vi "CreatePublicEvents.vi"(8 "error in (no error)":errorcluster, 11 "Setting Database":refnum<class "Setting Database.lvclass">) -> (0 "error out":errorcluster, 3 "Setting Database out":refnum<class "Setting Database.lvclass">)   [LabVIEW 2019, in "Setting Database.lvclass"]
doc: "---------------------------------------------------------------\nJKI State Machine Objects™\nhttp://jki.net/state-machine-objects/\nCopyright (C) 2005-2015, JKI <info@jki.net>\nALL RIGHTS RESERVEDJKI State Machine Objects (SMO) 1.0.0.4\nJKI - JKI\nCopyright (c) 2015, JKI"
uses:
  Setting Database.lvclass
  Typedefs/PublicEvents--Setting Database.NewActivePath.ctl
  Path Settings/Path Settings.lvclass
  Typedefs/PublicEvents--Setting Database.NewActiveRectangle.ctl
  Rectangle Settings/Rectangle Settings.lvclass
  Typedefs/PublicEvents--Setting Database.NewActiveFunnel.ctl
  Funnel Settings/Funnel Settings.lvclass
  Typedefs/PublicEvents--Setting Database.NewActiveDot.ctl
  Dot Settings/Dot Settings.lvclass
  Typedefs/PublicEvents--Setting Database.DotsUpdatedCheck.ctl
  Typedefs/PublicEvents--Setting Database.DotsUpdated.ctl
  Typedefs/PublicEvents--Setting Database.FunnelsUpdatedCheck.ctl
  Typedefs/PublicEvents--Setting Database.FunnelsUpdated.ctl
  Typedefs/PublicEvents--Setting Database.PathsUpdatedCheck.ctl
  Typedefs/PublicEvents--Setting Database.PathsUpdated.ctl
  Typedefs/PublicEvents--Setting Database.RectanglesUpdatedCheck.ctl
  Typedefs/PublicEvents--Setting Database.RectanglesUpdated.ctl
  Setting Database.lvclass/Setting Database.ctl
  <vilib>/JKI/JKI SMO/SMO/SMO.lvclass
panel:
  # "For instructions on how to use the JKI State Machine Objects, examples and video tutorials, visit:\nhttp://jki.net/state-machine-objects/\n\nJKI State Machine Objects™\nhttp://jki.net/state-machine-objects/\nCopyright (C) 2005-2015, JKI <info@jki.net>\nALL RIGHTS RESERVED"
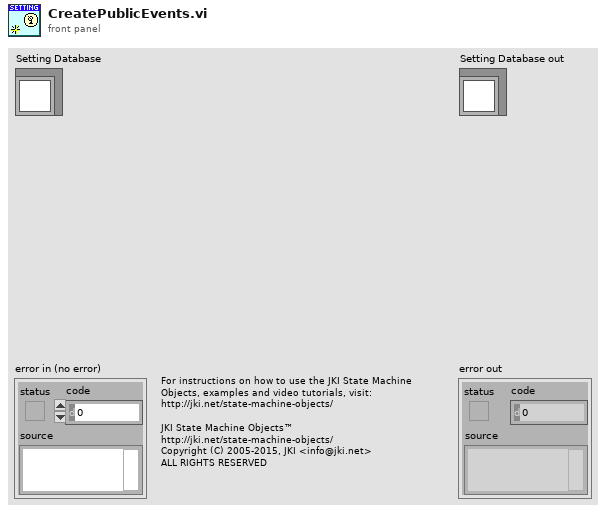
[diagram p1: front panel]
types:
  T1 = typedef "Setting Database.lvclass/PublicEvents--Setting Database.RectanglesUpdatedCheck.ctl" = cluster{"Read?":refnum<notifier>, "RectanglesUpdated":T2}
  T2 = typedef "Setting Database.lvclass/PublicEvents--Setting Database.RectanglesUpdated.ctl" = refnum<class "Rectangle Settings.lvclass">[]
  T3 = typedef "Setting Database.lvclass/PublicEvents--Setting Database.PathsUpdatedCheck.ctl" = cluster{"Read?":refnum<notifier>, "PathsUpdated":T4}
  T4 = typedef "Setting Database.lvclass/PublicEvents--Setting Database.PathsUpdated.ctl" = refnum<class "Path Settings.lvclass">[]
  T5 = typedef "Setting Database.lvclass/PublicEvents--Setting Database.FunnelsUpdatedCheck.ctl" = cluster{"Read?":refnum<notifier>, "FunnelsUpdated":T6}
  T6 = typedef "Setting Database.lvclass/PublicEvents--Setting Database.FunnelsUpdated.ctl" = refnum<class "Funnel Settings.lvclass">[]
  T7 = typedef "Setting Database.lvclass/PublicEvents--Setting Database.DotsUpdatedCheck.ctl" = cluster{"Read?":refnum<notifier>, "DotsUpdated":T8}
  T8 = typedef "Setting Database.lvclass/PublicEvents--Setting Database.DotsUpdated.ctl" = refnum<class "Dot Settings.lvclass">[]
  T9 = typedef "Setting Database.lvclass/PublicEvents--Setting Database.NewActiveDot.ctl" = refnum<class "Dot Settings.lvclass">
  T10 = typedef "Setting Database.lvclass/PublicEvents--Setting Database.NewActiveFunnel.ctl" = refnum<class "Funnel Settings.lvclass">
  T11 = typedef "Setting Database.lvclass/PublicEvents--Setting Database.NewActiveRectangle.ctl" = refnum<class "Rectangle Settings.lvclass">
  T12 = typedef "Setting Database.lvclass/PublicEvents--Setting Database.NewActivePath.ctl" = refnum<class "Path Settings.lvclass">
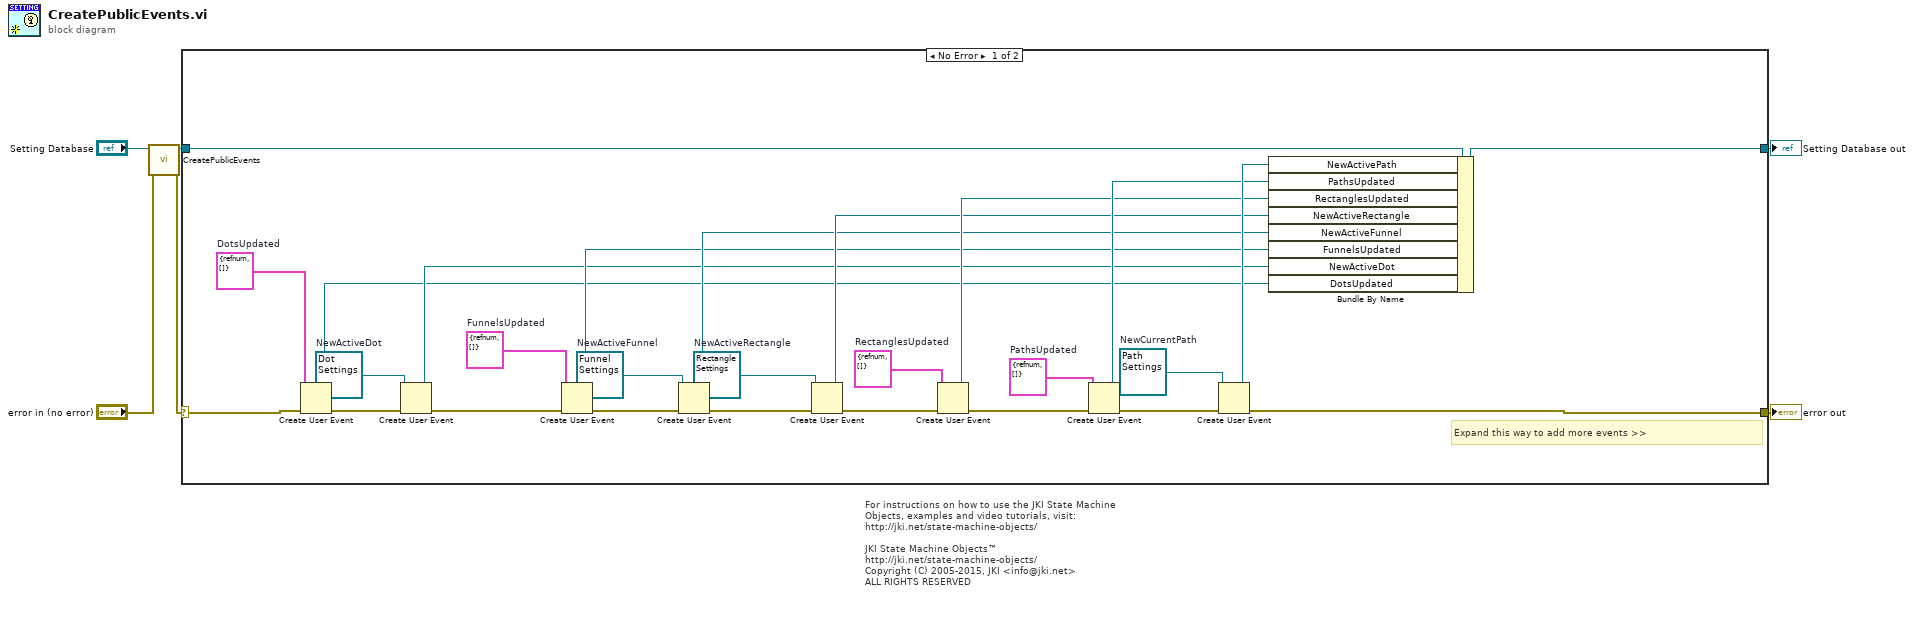
[diagram p0: block diagram]
diagram:
  # "For instructions on how to use the JKI State Machine Objects, examples and video tutorials, visit:\nhttp://jki.net/state-machine-objects/\n\nJKI State Machine Objects™\nhttp://jki.net/state-machine-objects/\nCopyright (C) 2005-2015, JKI <info@jki.net>\nALL RIGHTS RESERVED"
  n1 = call-parent "CreatePublicEvents.vi"("error in (no error)"="error in (no error)", "SMO"="Setting Database") -> ("error out"=w1:errorcluster, "SMO out"=w3:refnum<class "Setting Database.lvclass">)  [unwired: 8 in]
  n2 = case shown="No Error" w1 {
    selector: w1 -> [w32 w35]
    tunnel: [w30 w35] -> w5
    tunnel: [w31 w34] -> w6
    tunnel: w3 -> [w33 w34]
    frame No Error {
      w7 = T1 {"Read?"=refnum, "RectanglesUpdated"=[]}  # RectanglesUpdated
      w8 = T3 {"Read?"=refnum, "PathsUpdated"=[]}  # PathsUpdated
      w9 = T5 {"Read?"=refnum, "FunnelsUpdated"=[]}  # FunnelsUpdated
      w10 = T7 {"Read?"=refnum, "DotsUpdated"=[]}  # DotsUpdated
      w14 = T9 refnum  # NewActiveDot
      w19 = T10 refnum  # NewActiveFunnel
      w22 = T11 refnum  # NewActiveRectangle
      w29 = T12 refnum  # NewCurrentPath
      # "Expand this way to add more events >>"
      n3 = Create User Event(user event datatype=w10, error in=w32) -> (user event=w11:refnum<user-event>, error out=w12:errorcluster)
      n4 = Create User Event(user event datatype=w14, error in=w12) -> (user event=w13:refnum<user-event>, error out=w15:errorcluster)
      n5 = Create User Event(user event datatype=w9, error in=w15) -> (user event=w16:refnum<user-event>, error out=w17:errorcluster)
      n6 = Create User Event(user event datatype=w19, error in=w17) -> (user event=w18:refnum<user-event>, error out=w20:errorcluster)
      n7 = Create User Event(user event datatype=w22, error in=w20) -> (user event=w21:refnum<user-event>, error out=w23:errorcluster)
      n8 = Create User Event(user event datatype=w7, error in=w23) -> (user event=w24:refnum<user-event>, error out=w25:errorcluster)
      n9 = Create User Event(user event datatype=w8, error in=w25) -> (user event=w26:refnum<user-event>, error out=w27:errorcluster)
      n10 = Create User Event(user event datatype=w29, error in=w27) -> (user event=w28:refnum<user-event>, error out=w30:errorcluster)
      n11 = Bundle By Name(cluster=w33, "NewActivePath"=w28, "PathsUpdated"=w26, "RectanglesUpdated"=w24, "NewActiveRectangle"=w21, "NewActiveFunnel"=w18, "FunnelsUpdated"=w16, "NewActiveDot"=w13, "DotsUpdated"=w11) -> (w31:refnum<class "Setting Database.lvclass">)
    }
    frame Error {
    }
  }
  "error out" <- w5
  "Setting Database out" <- w6
